vi "Method3.vi"(8 "error in (no error)":errorcluster, 11 "Class 3 in":refnum<class "Class 3.lvclass">) -> (0 "error out":errorcluster, 3 "Class 3 out":refnum<class "Class 3.lvclass">)   [LabVIEW 2023, in "Class 3.lvclass"]
uses:
  Class 3.lvclass
  Class 3.lvclass/Class 3.ctl
panel:
  in  "message":string="Method 3, Class 3"
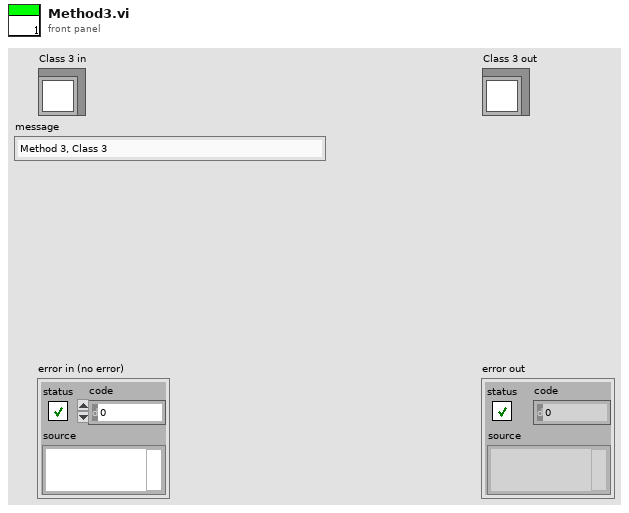
[diagram p1: front panel]
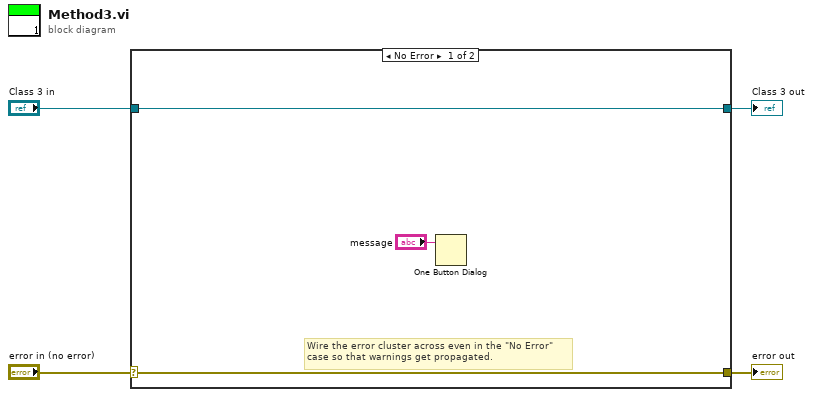
[diagram p0: block diagram]
diagram:
  n1 = case shown="No Error" "error in (no error)" {
    selector: "error in (no error)" -> [w6 w9]
    tunnel: [w6 w9] -> w3
    tunnel: [w7 w8] -> w1
    tunnel: "Class 3 in" -> [w7 w8]
    frame No Error {
      # "Wire the error cluster across even in the \"No Error\"\ncase so that warnings get propagated."
      n2 = One Button Dialog(message="message") -> ()  [unwired: 1 in, 1 out]
    }
    frame Error {
    }
  }
  "error out" <- w3
  "Class 3 out" <- w1
